vi "Teleop.vi"(10 "Match Info":T1={"Autonomous Elapsed Seconds"=0.0, "TeleOp Elapsed Seconds"=0.0, "Disabled Elapsed Seconds"=0.0, "Visited Autonomous"=FALSE, "Visited TeleOp"=FALSE, "Visited Disabled"=FALSE, "Autonomous Settings"={"Autonomous Style"=enum."Independent", "VI Refnum"=refnum}}, 11 "Call Context":T2) -> ()   [LabVIEW 2013]
doc: "This VI is called for each TeleOp packet received from the DS where the robot is not disabled. It is often used to read from the joysticks and update I/O or to update setpoints for timed control loops. It should complete and return within 20 milliseconds or it may miss DS packets."
uses:
  <vilib>/Rock Robotics/WPI/DriverStation/WPI_DriverStationDerivedRobotMode.ctl
  <vilib>/Rock Robotics/WPI/DriverStation/WPI_DriverStationMatch Info.ctl
  TeleopInstruction.ctl
  Robot Global Data.vi
  <vilib>/Rock Robotics/WPI/Joystick/WPI_JoystickGetSetRefNum.vi
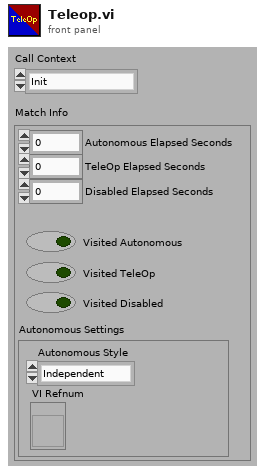
[diagram p1: front panel]
types:
  T1 = typedef "WPI_DriverStationMatch Info.ctl" = cluster{"Autonomous Elapsed Seconds":dbl, "TeleOp Elapsed Seconds":dbl, "Disabled Elapsed Seconds":dbl, "Visited Autonomous":bool, "Visited TeleOp":bool, "Visited Disabled":bool, "Autonomous Settings":cluster{"Autonomous Style":enum16{"Iterative", "Independent"}, "VI Refnum":refnum<vi>}}
  T2 = typedef "WPI_DriverStationDerivedRobotMode.ctl" = enum16{"Init", "Execute", "Stop"}
  T3 = typedef "TeleopInstruction.ctl" = cluster{"cDriveLeft":dbl, "cDriveRight":dbl, "cAutoDistance":bool, "cHalfDrive":bool, "cStraightDrive":bool, "cReverseDrive":bool, "cSonicShifter":bool, "cRoller":dbl, "cCollector":dbl, "cCatch":bool, "cCollectorWrap":bool, "cShooter":bool, "cClapper":bool, "cFiringPneumatic":bool, "cKickerPneumatic":bool, "cRollerPneumatic":bool}
  T4 = typedef "WPI_JoystickDevRef.ctl" = cluster{"Device":T5}
  T5 = typedef "WPI_JoystickDeviceEnum.ctl" = enum16{"USB 1", "USB 2", "USB 3", "USB 4", "Kinect 1", "Kinect 2"}
  T6 = typedef "WPI_JoystickButtonState.ctl" = cluster{"Button 1":bool, "Button 2":bool, "Button 3":bool, "Button 4":bool, "Button 5":bool, "Button 6":bool, "Button 7":bool, "Button 8":bool, "Button 9":bool, "Button 10":bool, "Button 11":bool, "Button 12":bool}
  T7 = cluster{"axis 1 (x)":dbl, "axis 2 (y)":dbl, "axis 3 (throttle)":dbl, "axis 4":dbl, "axis 5":dbl, "axis 6":dbl}
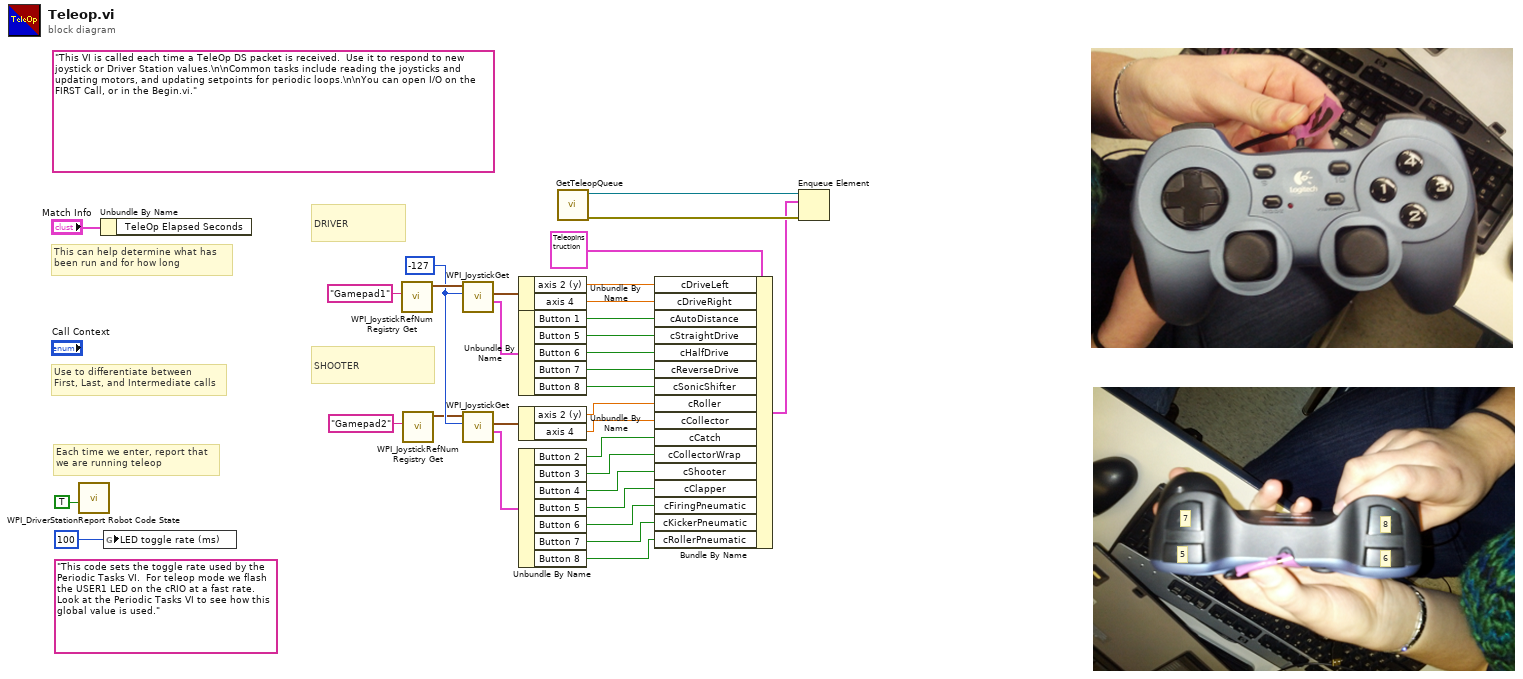
[diagram p0: block diagram]
diagram:
  w26 = i8 -127 ("Scaler")
  (unwired) "This code sets the toggle rate used by the Periodic Tasks VI.  For teleop mode we flash the USER1 LED on the cRIO at a fast rate.  Look at the Periodic Tasks VI to see how this global value is used."
  (unwired) "This VI is called each time a TeleOp DS packet is received.  Use it to respond to new joystick or Driver Station values.\n\nCommon tasks include reading the joysticks and updating motors, and updating setpoints for periodic loops.\n\nYou can open I/O on the FIRST Call, or in the Begin.vi."
  # "SHOOTER"
  # "DRIVER"
  # "5"
  # "7"
  # "6"
  # "8"
  # "Each time we enter, report that\nwe are running teleop"
  # "Use to differentiate between\nFirst, Last, and Intermediate calls"
  # "This can help determine what has\nbeen run and for how long"
  n1 = call <vilib>:"WPI_DriverStationReport Robot Code State.vi"("TeleOp"=TRUE ("Autonomous")) -> ()  [unwired: 10 in, 1 out]
  n2 = Unbundle By Name("Match Info") -> ()  [unwired: 1 out]
  n3 = global write "Robot Global Data.vi" "LED toggle rate (ms)"(u32 100 ("LED ms toggle rate")) -> ()
  n4 = call <vilib>:"WPI_JoystickRefNum Registry Get.vi"("refnum name"="Gamepad1") -> ("JoystickDevRef"=w27:T4)  [unwired: 9 in, 1 out]
  n5 = call <vilib>:"WPI_JoystickRefNum Registry Get.vi"("refnum name"="Gamepad2") -> ("JoystickDevRef"=w25:T4)  [unwired: 9 in, 1 out]
  n6 = call <vilib>:"WPI_JoystickGet.vi"("Scaler"=w26, "JoystickDevRef"=w27) -> ("Buttons"=w23:T6, "Axes"=w24:T7)  [unwired: 3 in, 1 out]
  n7 = call <vilib>:"WPI_JoystickGet.vi"("Scaler"=w26, "JoystickDevRef"=w25) -> ("Buttons"=w21:T6, "Axes"=w22:T7)  [unwired: 3 in, 1 out]
  n8 = Unbundle By Name(w24) -> ("axis 2 (y)"=w16:dbl, "axis 4"=w15:dbl)
  n9 = Unbundle By Name(w23) -> ("Button 1"=w1:bool, "Button 5"=w2:bool, "Button 6"=w14:bool, "Button 7"=w13:bool, "Button 8"=w12:bool)
  n10 = Unbundle By Name(w22) -> ("axis 2 (y)"=w6:dbl, "axis 4"=w7:dbl)
  n11 = Unbundle By Name(w21) -> ("Button 2"=w3:bool, "Button 3"=w4:bool, "Button 4"=w5:bool, "Button 5"=w8:bool, "Button 6"=w11:bool, "Button 7"=w10:bool, "Button 8"=w9:bool)
  n12 = call "GetTeleopQueue.vi"() -> ("error out"=w19:errorcluster, "queue out"=w20:refnum<queue>)  [unwired: 10 in]
  n13 = Bundle By Name(cluster=T3 {"cDriveLeft"=0.0, "cDriveRight"=0.0, "cAutoDistance"=FALSE, "cHalfDrive"=FALSE, "cStraightDrive"=FALSE, "cReverseDrive"=FALSE, "cSonicShifter"=FALSE, "cRoller"=0.0, "cCollector"=0.0, "cCatch"=FALSE, "cCollectorWrap"=FALSE, "cShooter"=FALSE, "cClapper"=FALSE, "cFiringPneumatic"=FALSE, "cKickerPneumatic"=FALSE, "cRollerPneumatic"=FALSE} ("TeleopInstruction"), "cDriveLeft"=w16, "cDriveRight"=w15, "cAutoDistance"=w1, "cStraightDrive"=w2, "cHalfDrive"=w14, "cReverseDrive"=w13, "cSonicShifter"=w12, "cRoller"=w6, "cCollector"=w7, "cCatch"=w3, "cCollectorWrap"=w4, "cShooter"=w5, "cClapper"=w8, "cFiringPneumatic"=w11, "cKickerPneumatic"=w10, "cRollerPneumatic"=w9) -> (w17:T3)
  n14 = Enqueue Element(queue=w20, element=w17, error in (no error)=w19) -> ()  [unwired: 1 in, 3 out]
